vi "Client.vi"() -> ()   [LabVIEW 2014]
panel:
  in  "Stop Button":bool
  in  "My Tank Value":dbl(slide) scale=0.0..10.0
  # "Destributed Systems\n(Client)"
  # "My Tank"
  # "Exit"
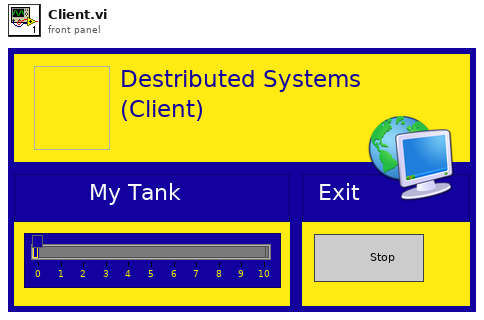
[diagram p1: front panel]
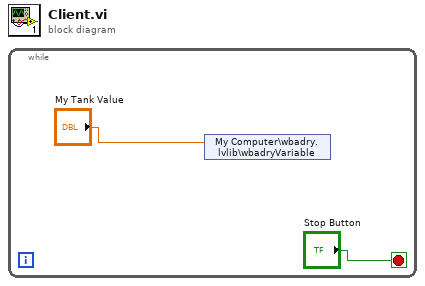
[diagram p0: block diagram]
diagram:
  n1 = while {
    stop <- "Stop Button" stop-if-true
    n2 = shared-variable "My Computer\\wbadry.lvlib\\wbadryVariable"("My Tank Value") -> ()  [unwired: 1 in, 1 out]
  }
